vi "niRFUtil WFM Threshold Array.vi"(2 "Threshold":sgl, 3 "Array In":T1 min=0 max=127 format="%.2f") -> (0 "Below Threshold":T1 min=0 max=127 format="%.2f", 1 "Above Threshold":T1 min=0 max=127 format="%.2f")   [LabVIEW 2015, in "niRFUtil.lvlib"]
doc: "(c) Copyright 2006, National Instruments, Inc. This VI may not be duplicated, sold, or distributed without written consent from National Instruments."
uses:
  niRFUtil.lvlib
  Includes/niRFUtil INC Real Array.ctl
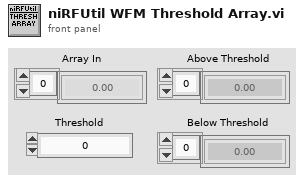
[diagram p1: front panel]
types:
  T1 = typedef "niRFUtil.lvlib/niRFUtil INC Real Array.ctl" = sgl[]
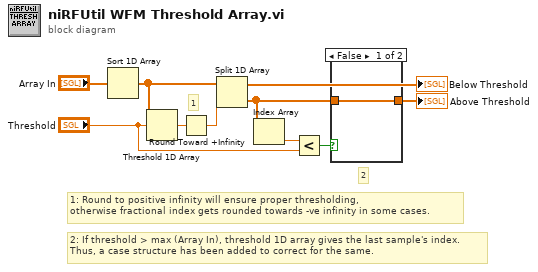
[diagram p0: block diagram]
diagram:
  # "2"
  # "1"
  # "2: If threshold > max (Array In), threshold 1D array gives the last sample's index.\nThus, a case structure has been added to correct for the same."
  # "1: Round to positive infinity will ensure proper thresholding, \notherwise fractional index gets rounded towards -ve infinity in some cases."
  n1 = Sort 1D Array(array="Array In") -> (sorted array=w9:T1)
  n2 = Threshold 1D Array(2:"Threshold", 3:w9) -> (0:w7:sgl)  [unwired: 1 in]
  n3 = Round Toward +Infinity(x=w7) -> (ceil(x): smallest int >= x=w6:sgl)
  n4 = Split 1D Array(array=w9, index=w6) -> (first subarray=→"Below Threshold":T1, second subarray=w2:T1)
  n5 = Index Array(array=w2) -> (element=w5:sgl)  [unwired: 1 in]
  n6 = Less?(x=w5, y="Threshold") -> (x < y?=w3:bool)
  n7 = case shown="False" w3 {
    tunnel: w2 -> [w11 _]
    tunnel: [w11 _] -> w1
    frame False {
    }
    frame True {
    }
  }
  "Above Threshold" <- w1
